vi "ChapR Button Translate.vi"(9 "B2":u8, 10 "B1":u8) -> (2 "B":u16)   [LabVIEW 2013]
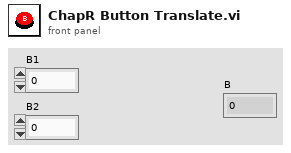
[diagram p1: front panel]
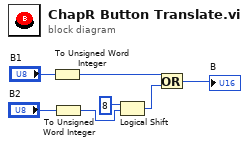
[diagram p0: block diagram]
diagram:
  n1 = To Unsigned Word Integer(number="B1") -> (unsigned 16bit integer=w3:u16)
  n2 = To Unsigned Word Integer(number="B2") -> (unsigned 16bit integer=w5:u16)
  n3 = Logical Shift(y=i16 8, x=w5) -> (x << y=w2:u16)
  n4 = Or(x=w3, y=w2) -> (x .or. y?=→"B":u16)
